vi "Example 4 - Primitive Functions (Part 2).vi"   [LabVIEW 2015]
uses:
  library/Scripting.lvlib
types:
  T1 = cluster{"Boolean":bool, "Number":dbl, "String":string}
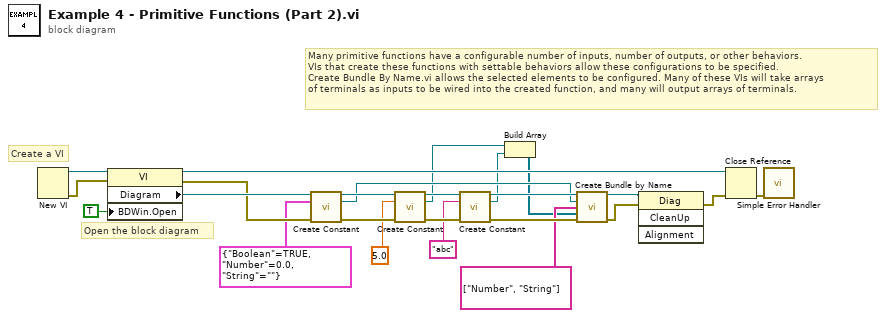
[diagram p0: block diagram]
diagram:
  # "Many primitive functions have a configurable number of inputs, number of outputs, or other behaviors.\nVIs that create these functions with settable behaviors allow these configurations to be specified.\nCreate Bundle By Name.vi allows the selected elements to be configured. Many of these VIs will take arrays\nof terminals as inputs to be wired into the created function, and many will output arrays of terminals."
  # "Open the block diagram"
  # "Create a VI"
  n1 = New VI() -> (0:w19:errorcluster, 3:w20:refnum<vi>)  [unwired: 7 in]
  n2 = property class="VI"(reference=w20, error in=w19, "BDWin.Open"=TRUE ("Block Diagram Window:Open")) -> (reference out=w21:refnum<vi>, error out=w17:errorcluster, "Diagram"=w18:refnum<vi>)
  n3 = call "Create Constant.vi"("Diagram in"=w18, "Type"=T1 {"Boolean"=TRUE, "Number"=0.0, "String"=""}, "error in (no error)"=w17) -> ("Diagram out"=w15:refnum<vi>, "Terminal"=w7:refnum<vi>, "error out"=w14:errorcluster)  [unwired: 10 in]
  n4 = call "Create Constant.vi"("Diagram in"=w15, "Type"=5.0, "error in (no error)"=w14) -> ("Diagram out"=w13:refnum<vi>, "Terminal"=w3:refnum<vi>, "error out"=w12:errorcluster)  [unwired: 10 in]
  n5 = call "Create Constant.vi"("Diagram in"=w13, "Type"="abc", "error in (no error)"=w12) -> ("Diagram out"=w9:refnum<vi>, "Terminal"=w2:refnum<vi>, "error out"=w8:errorcluster)  [unwired: 10 in]
  n6 = Build Array(w3, w2) -> (w1:refnum<vi>[])
  n7 = call "Create Bundle by Name.vi"("Diagram in"=w9, "input cluster"=w7, "Element Names"=string[] ["Number", "String"], "Inputs"=w1, "error in (no error)"=w8) -> ("Diagram out"=w4:refnum<vi>, "error out"=w5:errorcluster)  [unwired: 8 in, 1 out]
  n8 = invoke class="Diag" method="CleanUp"(reference=w4, error in=w5) -> (error out=w23:errorcluster)  [unwired: 2 in, 3 out]
  n9 = Close Reference(reference=w21, error in (no error)=w23) -> (error out=w22:errorcluster)
  n10 = call <vilib>:"Simple Error Handler.vi"("error in (no error)"=w22) -> ()  [unwired: 4 in, 5 out]
